vi "COM_ParseCommand.vi"(8 "error in":errorcluster, 11 "Message in":string) -> (0 "error out":errorcluster, 2 "Parameters":string, 3 "Command":string)   [LabVIEW 2020, in "hse-network.lvlib"]
doc: "(v0.2.1b; 2017-08-14 16:44)\n\n\n\n____\nHAMPEL SOFTWARE ENGINEERING v3.8.0 (2023-12-18 14:41)"
uses:
  hse-network.lvlib
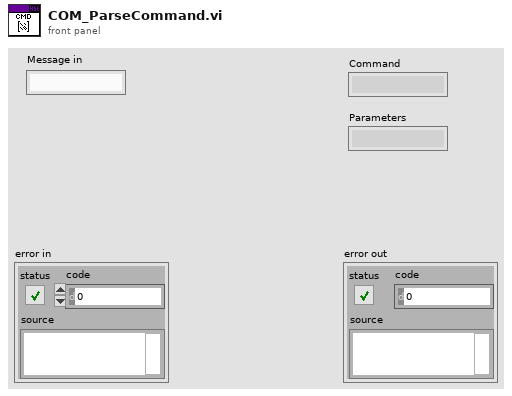
[diagram p1: front panel]
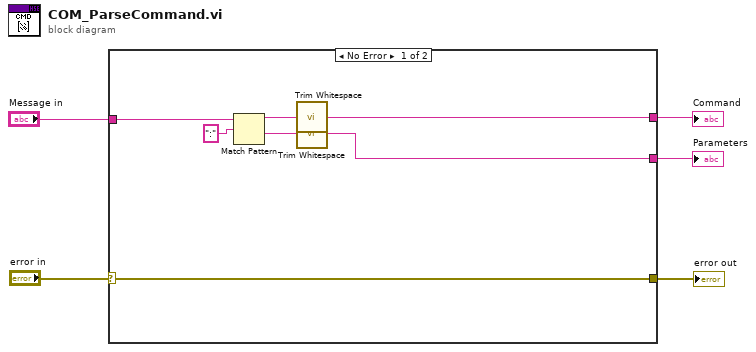
[diagram p0: block diagram]
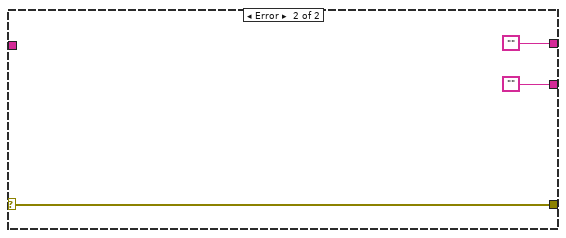
[diagram p2: hidden frame]
diagram:
  n1 = case shown="No Error" "error in" {
    selector: "error in" -> [w8 w15]
    tunnel: [w8 w15] -> w4
    tunnel: [w7 ""] -> w3
    tunnel: [w6 ""] -> w2
    tunnel: "Message in" -> [w11 _]
    frame No Error {
      n2 = Match Pattern(string=w11, regular expression=":") -> (before substring=w10:string, after substring=w9:string)  [unwired: 1 in, 2 out]
      n3 = call <vilib>:"Trim Whitespace.vi"("string"=w10) -> ("trimmed string"=w7:string)  [unwired: 1 in]
      n4 = call <vilib>:"Trim Whitespace.vi"("string"=w9) -> ("trimmed string"=w6:string)  [unwired: 1 in]
    }
    frame Error {
    }
  }
  "error out" <- w4
  "Parameters" <- w2
  "Command" <- w3
